vi "Pen Attributes And Image subsetting.vi"() -> ()   [LabVIEW 2023]
doc: "The picture control can be used as a drawing interface for users. The main features that are used in this example are the Pen Width and Style attributes and the Subsetting feature. Subsetting is the ability to take a rectangular subset of any image and draw a new image."
uses:
  <vilib>/Utility/cursorutil.llb/Set Cursor (Icon Pict).vi
panel:
  in  "Clear":bool
  in  "Pen Color":u32(colorbox)=15671808
  in  "Stop":bool
  in  "Operation":u16(ring)=1 items=["Draw Scattered Points", "Draw Free-form Line", "Draw Straight Line", "Draw Rectangle", "Select Subset"]
  out "Subset":picture
  in  "Select Pen Attributes":T1={"Width"=6, "Style"=enum."Solid"}
  out "Picture":picture
  # "Overview: Demonstrates the 2D Picture as a drawing interface.\nInstructions:\n1. Run the VI.\n2. Choose the Operation you want to perform.\n3. Move the mouse over the Picture and click-drag to draw on it.  If you chose Select Subset, a box will be used to define the area to be copied into the Subset picture.\n4. Change the pen color by clicking the Pen Color box.\n5. Clear the picture with the Clear button.\n6. Click Stop to stop the VI."
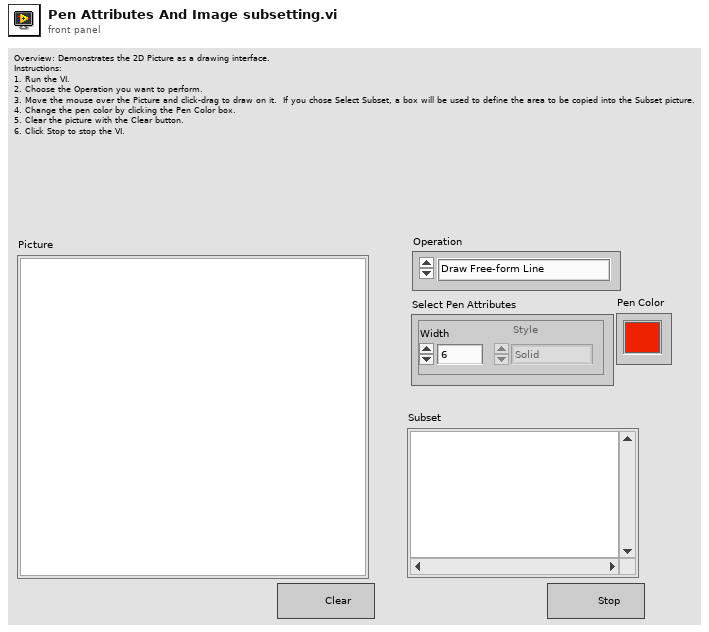
[diagram p1: front panel]
types:
  T1 = cluster{"Width":u16, "Style":enum32{"Solid", "Dash", "Dot", "DashDot", "DashDotDot"}}
  T2 = enum32{"Solid", "Dash", "Dot", "DashDot", "DashDotDot"}
  T3 = enum8{"Enabled", "Disabled", "Disabled and Grayed Out"}
  T4 = typedef "LVMouseTypeDef.ctl" = cluster{"Mouse Position":cluster{"X":i32, "Y":i32}, "Mouse Modifiers":cluster{"Button Down":bool, "Shift Mod":bool, "Menu Mod":bool, "Option Mod":bool}}
  T5 = typedef "imagedata.ctl" = cluster{"image type":i32, "image depth":i32, "image":u8[], "mask":u8[], "colors":u32[], "Rectangle":cluster{"left":i16, "top":i16, "right":i16, "bottom":i16}}
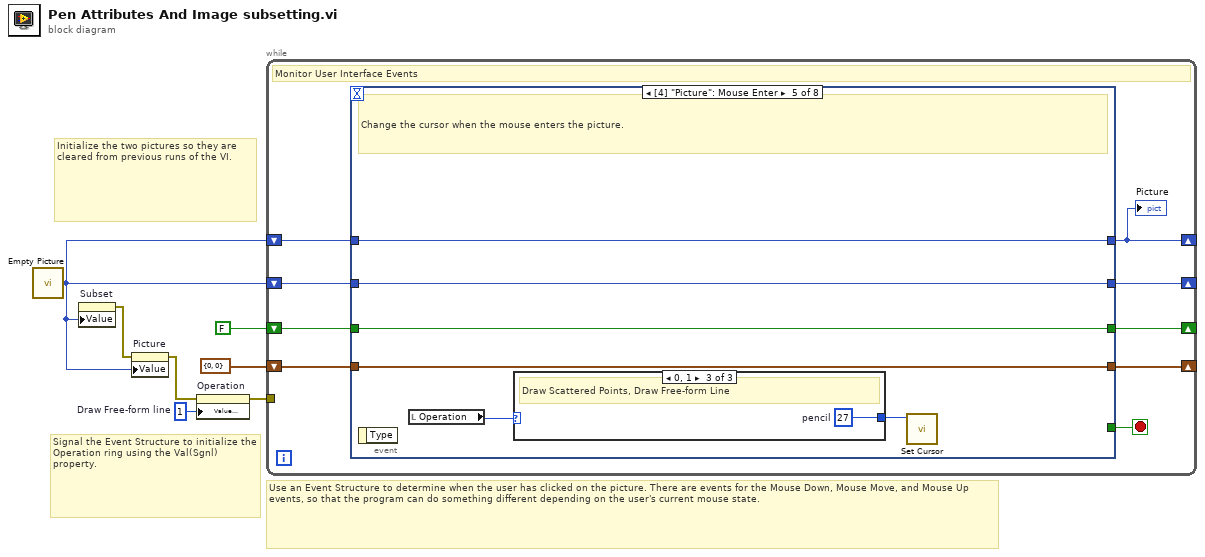
[diagram p0: block diagram]
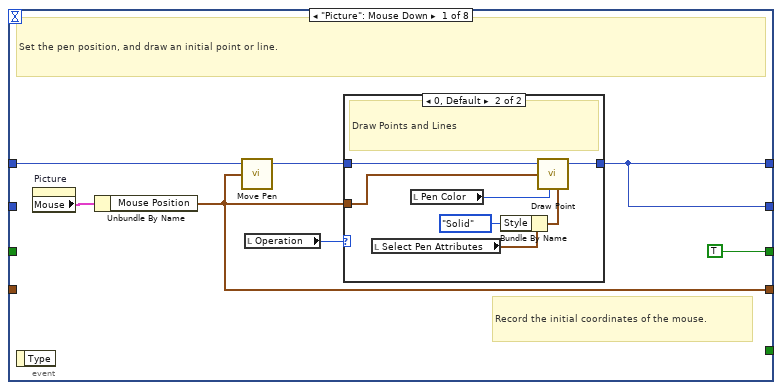
[diagram p2: hidden frame]
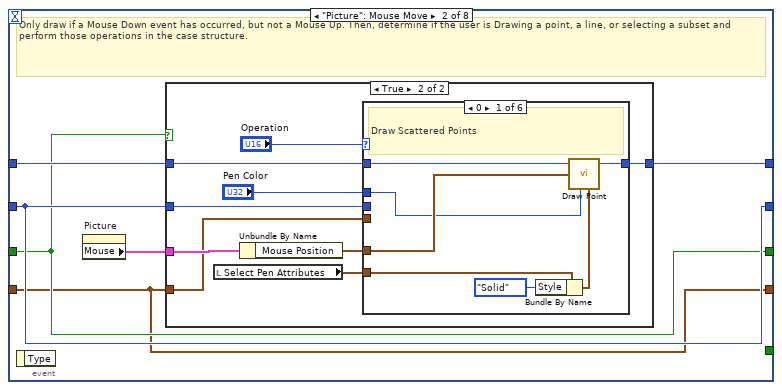
[diagram p4: hidden frame]
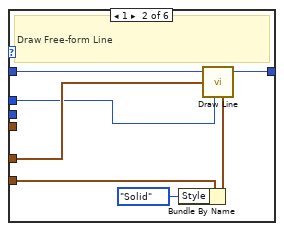
[diagram p6: hidden frame]
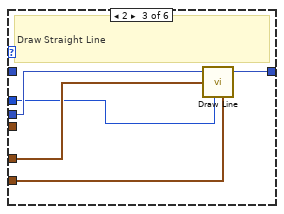
[diagram p7: hidden frame]
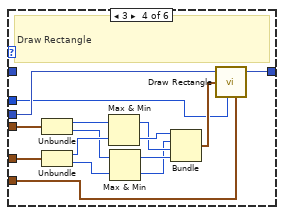
[diagram p8: hidden frame]
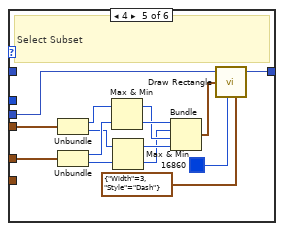
[diagram p9: hidden frame]
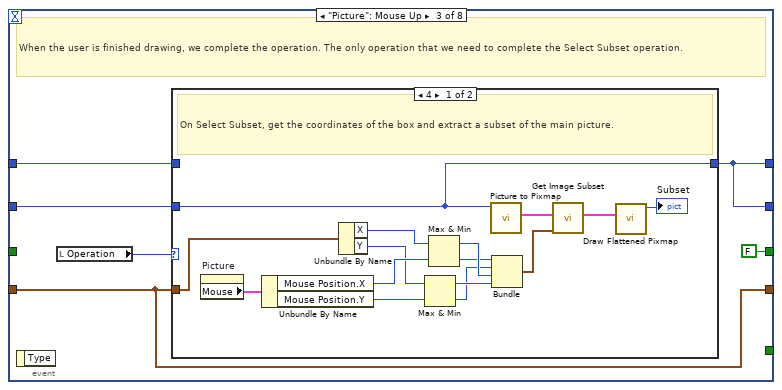
[diagram p11: hidden frame]
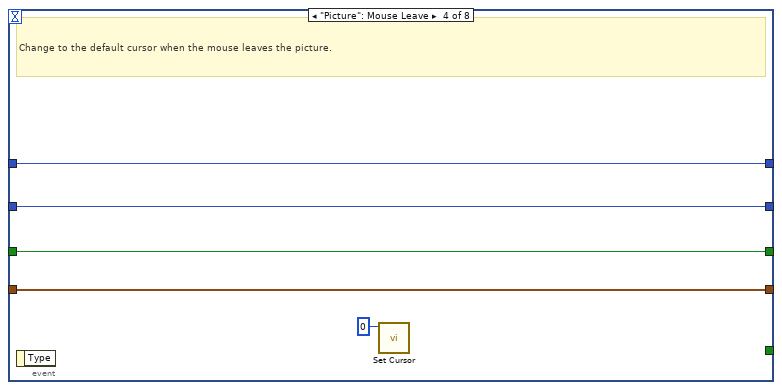
[diagram p13: hidden frame]
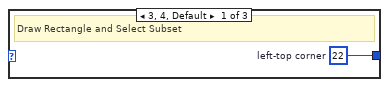
[diagram p14: hidden frame]
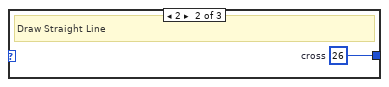
[diagram p15: hidden frame]
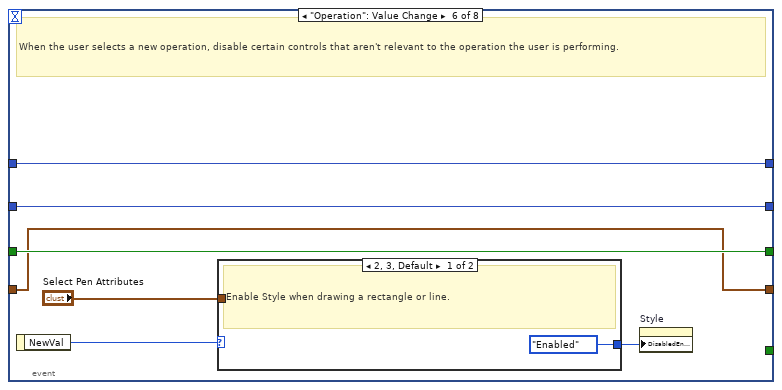
[diagram p16: hidden frame]
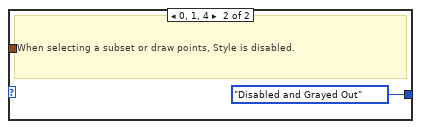
[diagram p17: hidden frame]
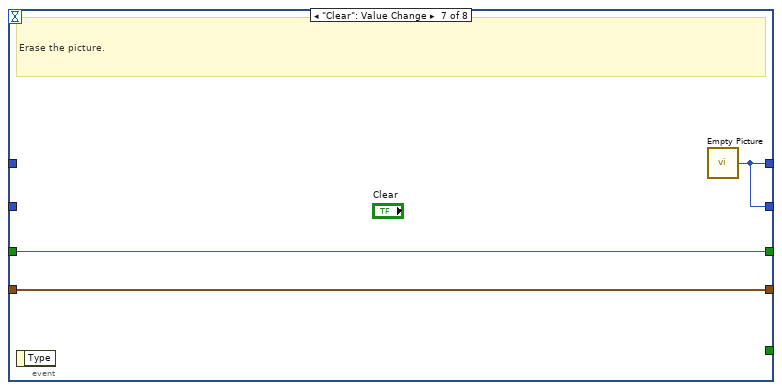
[diagram p18: hidden frame]
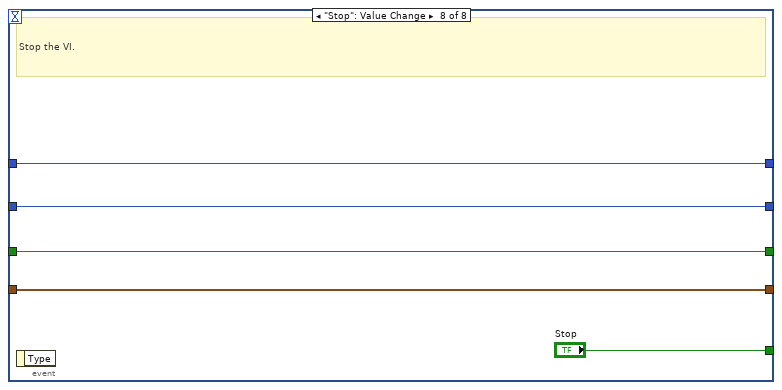
[diagram p19: hidden frame]
diagram:
  w4 = u16 1  # Draw Free-form line
  # "Use an Event Structure to determine when the user has clicked on the picture. There are events for the Mouse Down, Mouse Move, and Mouse Up events, so that the program can do something different depending on the user's current mouse state."
  # "Signal the Event Structure to initialize the Operation ring using the Val(Sgnl) property."
  # "Initialize the two pictures so they are cleared from previous runs of the VI."
  n1 = call "Empty Picture"() -> ("empty picture"=w3:picture)
  n2 = property on="Subset" class="Pict"("Value"=w3) -> (error out=w5:errorcluster)  [unwired: 2 in, 1 out]
  n3 = property on="Picture" class="Pict"(error in=w5, "Value"=w3) -> (error out=w6:errorcluster)  [unwired: 1 in, 1 out]
  n4 = property on="Operation" class="Ring (strict)"(error in=w6, "Value (Signaling)"=w4) -> (error out=w7:errorcluster)  [unwired: 1 in, 1 out]
  n5 = while {
    shift-right: [w15] -> _
    shift-left: w3 -> [w14]
    tunnel: w7 -> [_]
    shift-right: [w12] -> _
    shift-left: w3 -> [w13]
    shift-right: [w10] -> _
    shift-left: FALSE -> [w11]
    shift-right: [w8] -> _
    shift-left: cluster{"X":i32, "Y":i32} {"X"=0, "Y"=0} ("Mouse Position") -> [w9]
    stop <- w16 stop-if-true
    # "Monitor User Interface Events"
    n6 = event shown="[4] \"Picture\": Mouse Enter" {
      selector: _ -> [_ _ _ _ _ _ _ _]
      dyn-events: _ -> [_ _ _ _ _ _ _ _]
      timeout: _ -> [_ _ _ _ _ _ _ _]
      tunnel: [_ _ _ _ _ _ _ "Stop"] -> w16
      tunnel: [w20 w36 w100 w123 w129 w139 w145 w149] -> w12
      tunnel: w13 -> [w22 w35 w102 w123 w129 w139 _ w149]
      tunnel: [w20 w34 w100 w124 w130 w138 w145 w148] -> w15
      tunnel: w14 -> [_ w34 w101 w124 w130 w138 _ w148]
      tunnel: w11 -> [_ w33 _ w121 w126 w135 w144 w147]
      tunnel: [TRUE w33 FALSE w121 w126 w135 w144 w147] -> w10
      tunnel: w9 -> [_ w32 w98 w120 w125 w134 w143 w146]
      tunnel: [w17 w32 w98 w120 w125 w134 w143 w146] -> w8
      event "Picture": Mouse Down {
        # "Record the initial coordinates of the mouse."
        # "Set the pen position, and draw an initial point or line."
        n7 = event-data() -> ()  [unwired: 1 in, 1 out]
        n8 = property on="Picture" class="Pict"() -> ("Mouse"=w23:T4)  [unwired: 2 in, 2 out]
        n9 = Unbundle By Name(w23) -> ("Mouse Position"=w17:cluster{"X":i32, "Y":i32})
        n10 = call <vilib>:"Move Pen.vi"("new position"=w17, "picture"=w22) -> ("new picture"=w21:picture)  [unwired: 3 in]
        n11 = local read "Operation"() -> (w19:u16)
        n12 = case shown="0, Default" w19 {
          tunnel: w21 -> [w24 w31]
          tunnel: [w24 w30] -> w20
          tunnel: w17 -> [_ w29]
          frame 3, 4 {
            # "Draw Rectangles"
          }
          frame 0, Default {
            # "Draw Points and Lines"
            n13 = local read "Select Pen Attributes"() -> (w26:T1)
            n14 = local read "Pen Color"() -> (w28:u32)
            n15 = Bundle By Name(cluster=w26, "Style"=T2."Solid") -> (w25:T1)
            n16 = call <vilib>:"Draw Point.vi"("picture"=w31, "point(x,y)"=w29, "color(black)"=w28, "pen"=w25) -> ("new picture"=w30:picture)  [unwired: 5 in]
          }
        }
      }
      event "Picture": Mouse Move {
        # "Only draw if a Mouse Down event has occurred, but not a Mouse Up. Then, determine if the user is Drawing a point, a line, or selecting a subset and perform those operations in the case structure."
        n17 = event-data() -> ()  [unwired: 1 in, 1 out]
        n18 = property on="Picture" class="Pict"() -> ("Mouse"=w37:T4)  [unwired: 2 in, 2 out]
        n19 = case shown="True" w33 {
          tunnel: w35 -> [w38 w46]
          tunnel: w37 -> [_ w45]
          tunnel: [w38 w43] -> w36
          tunnel: w34 -> [_ w42]
          tunnel: w32 -> [_ w41]
          frame False {
          }
          frame True {
            n20 = local read "Select Pen Attributes"() -> (w40:T1)
            n21 = Unbundle By Name(w45) -> ("Mouse Position"=w44:cluster{"X":i32, "Y":i32})
            n22 = case shown="0" "Operation" {
              tunnel: w46 -> [w52 w59 _ _ _ w97]
              tunnel: w41 -> [_ _ _ w80 w95 _]
              tunnel: w44 -> [w53 w60 w65 w81 w96 _]
              tunnel: [w54 w61 w66 w78 w93 w97] -> w43
              tunnel: w42 -> [_ _ w64 w70 w92 _]
              tunnel: w40 -> [w49 w56 w63 w69 _ _]
              tunnel: "Pen Color" -> [w48 w55 w62 w68 _ _]
              frame 0 {
                # "Draw Scattered Points"
                n23 = Bundle By Name(cluster=w49, "Style"=T2."Solid") -> (w51:T1)
                n24 = call <vilib>:"Draw Point.vi"("picture"=w52, "point(x,y)"=w53, "color(black)"=w48, "pen"=w51) -> ("new picture"=w54:picture)  [unwired: 5 in]
              }
              frame 1 {
                # "Draw Free-form Line"
                n25 = Bundle By Name(cluster=w56, "Style"=T2."Solid") -> (w57:T1)
                n26 = call <vilib>:"Draw Line.vi"("picture"=w59, "end point"=w60, "color(black)"=w55, "pen"=w57) -> ("new picture"=w61:picture)  [unwired: 5 in]
              }
              frame 2 {
                # "Draw Straight Line"
                n27 = call <vilib>:"Draw Line.vi"("picture"=w64, "end point"=w65, "color(black)"=w62, "pen"=w63) -> ("new picture"=w66:picture)  [unwired: 5 in]
              }
              frame 3 {
                # "Draw Rectangle"
                n28 = Unbundle(w80) -> ("X"=w77:i32, "Y"=w67:i32)
                n29 = Unbundle(w81) -> ("X"=w76:i32, "Y"=w73:i32)
                n30 = Max & Min(x=w77, y=w76) -> (max(x,y)=w74:i32, min(x,y)=w75:i32)
                n31 = Max & Min(x=w67, y=w73) -> (max(x,y)=w72:i32, min(x,y)=w71:i32)
                n32 = Bundle(w75, w71, w74, w72) -> (w79:cluster{i32, i32, i32, i32})  [unwired: 1 in]
                n33 = call <vilib>:"Draw Rectangle.vi"("picture"=w70, "rect"=w79, "color(black)"=w68, "pen"=w69) -> ("new picture"=w78:picture)  [unwired: 5 in]
              }
              frame 4 {
                # "Select Subset"
                n34 = Unbundle(w95) -> ("X"=w91:i32, "Y"=w87:i32)
                n35 = Unbundle(w96) -> ("X"=w90:i32, "Y"=w86:i32)
                n36 = Max & Min(x=w91, y=w90) -> (max(x,y)=w88:i32, min(x,y)=w89:i32)
                n37 = Max & Min(x=w87, y=w86) -> (max(x,y)=w85:i32, min(x,y)=w84:i32)
                n38 = Bundle(w89, w84, w88, w85) -> (w94:cluster{i32, i32, i32, i32})  [unwired: 1 in]
                n39 = call <vilib>:"Draw Rectangle.vi"("picture"=w92, "rect"=w94, "color(black)"=u32 16860, "pen"=T1 {"Width"=3, "Style"=enum."Dash"} ("Select Pen Attributes")) -> ("new picture"=w93:picture)  [unwired: 5 in]
              }
              frame Default {
                # "Operation not defined - do nothing."
              }
            }
          }
        }
      }
      event "Picture": Mouse Up {
        # "When the user is finished drawing, we complete the operation. The only operation that we need to complete the Select Subset operation."
        n40 = event-data() -> ()  [unwired: 1 in, 1 out]
        n41 = local read "Operation"() -> (w103:u16)
        n42 = case shown="4" w103 {
          tunnel: w102 -> [_ w119]
          tunnel: [w113 w119] -> w100
          tunnel: w101 -> [w113 _]
          tunnel: w98 -> [w104 _]
          frame 4 {
            # "On Select Subset, get the coordinates of the box and extract a subset of the main picture."
            n43 = property on="Picture" class="Pict"() -> ("Mouse"=w117:T4)  [unwired: 2 in, 2 out]
            n44 = Unbundle By Name(w117) -> ("Mouse Position.X"=w107:i32, "Mouse Position.Y"=w105:i32)
            n45 = Unbundle By Name(w104) -> ("X"=w108:i32, "Y"=w106:i32)
            n46 = Max & Min(x=w106, y=w105) -> (max(x,y)=w110:i32, min(x,y)=w109:i32)
            n47 = Max & Min(x=w108, y=w107) -> (max(x,y)=w112:i32, min(x,y)=w111:i32)
            n48 = call <vilib>:"Picture to Pixmap.vi"("picture"=w113) -> ("image data"=w118:T5)  [unwired: 9 in, 1 out]
            n49 = Bundle(w111, w109, w112, w110) -> (w116:cluster{i32, i32, i32, i32})  [unwired: 1 in]
            n50 = call <vilib>:"Get Image Subset.vi"("subset rect"=w116, "image data"=w118) -> ("image subset"=w115:T5)  [unwired: 4 in, 1 out]
            n51 = call <vilib>:"Draw Flattened Pixmap.vi"("image data"=w115) -> ("new picture"=→"Subset":picture)  [unwired: 8 in]
          }
          frame Default {
            # "Do nothing on mouse up for anything other than Select Subset."
          }
        }
      }
      event "Picture": Mouse Leave {
        # "Change to the default cursor when the mouse leaves the picture."
        n52 = event-data() -> ()  [unwired: 1 in, 1 out]
        n53 = call-poly <vilib>:"Set Cursor.vi"("icon"=u16 0) -> ()  [unwired: 9 in, 2 out]
      }
      event "Picture": Mouse Enter {
        # "Change the cursor when the mouse enters the picture."
        n54 = event-data() -> ()  [unwired: 1 in, 1 out]
        n55 = local read "Operation"() -> (w127:u16)
        n56 = case shown="0, 1" w127 {
          tunnel: [w131 w132 w133] -> w128
          frame 3, 4, Default {
            w131 = u16 22  # left-top corner
            # "Draw Rectangle and Select Subset"
          }
          frame 2 {
            w132 = u16 26  # cross
            # "Draw Straight Line"
          }
          frame 0, 1 {
            w133 = u16 27  # pencil
            # "Draw Scattered Points, Draw Free-form Line"
          }
        }
        n57 = call-poly <vilib>:"Set Cursor.vi"("icon"=w128) -> ()  [unwired: 9 in, 2 out]
      }
      event "Operation": Value Change {
        # "When the user selects a new operation, disable certain controls that aren't relevant to the operation the user is performing."
        n58 = event-data() -> ("NewVal"=w140:u16)  [unwired: 1 in]
        n59 = case shown="2, 3, Default" w140 {
          tunnel: "Select Pen Attributes" -> [_ _]
          tunnel: [T3."Enabled" ("Disabled") T3."Disabled and Grayed Out" ("Disabled")] -> w136
          frame 2, 3, Default {
            # "Enable Style when drawing a rectangle or line."
          }
          frame 0, 1, 4 {
            # "When selecting a subset or draw points, Style is disabled."
          }
        }
        n60 = property on="Style" class="Enum (strict)"("DisabledEnum"=w136) -> ()  [unwired: 2 in, 2 out]
      }
      event "Clear": Value Change {
        # "Erase the picture."
        n61 = event-data() -> ()  [unwired: 1 in, 1 out]
        n62 = call "Empty Picture"() -> ("empty picture"=w145:picture)
      }
      event "Stop": Value Change {
        # "Stop the VI."
        n63 = event-data() -> ()  [unwired: 1 in, 1 out]
      }
    }
    "Picture" <- w12
  }
